vi "Initialise Listbox.vi"(8 "error in (no error)":errorcluster, 11 "MulticolumnListbox in":refnum<vi>) -> (0 "error out":errorcluster)   [LabVIEW 2016, in "Assert API Components.lvlib" / "Assert Display.lvlib" / "Main Display.lvlib" / "Main Display.lvclass"]
uses:
  Main Display.lvclass
  <vilib>/Utility/miscctls.llb/LVRowAndColumnTypeDef.ctl
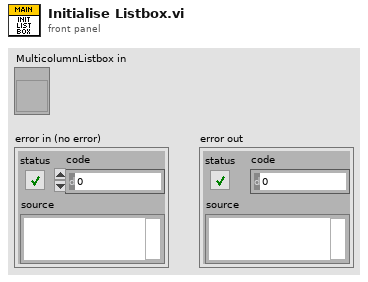
[diagram p1: front panel]
types:
  T1 = typedef "LVRowAndColumnTypeDef.ctl" = cluster{"Row":i32, "Column":i32}
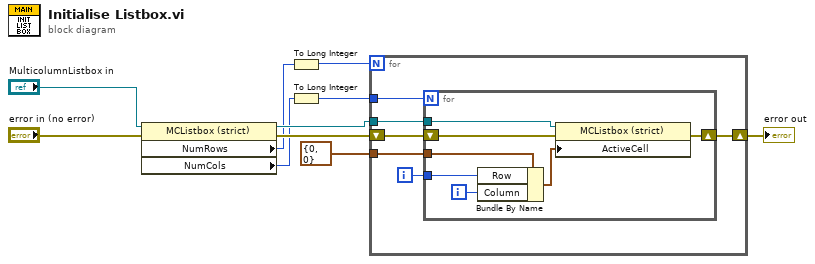
[diagram p0: block diagram]
diagram:
  n1 = property class="MCListbox (strict)"(reference="MulticolumnListbox in", error in="error in (no error)") -> (reference out=w6:refnum<vi>, error out=w9:errorcluster, "NumRows"=w4:u32, "NumCols"=w3:u32)
  n2 = To Long Integer(number=w4) -> (32bit integer=w2:i32)
  n3 = To Long Integer(number=w3) -> (32bit integer=w1:i32)
  n4 = for {
    N: w2 -> [_]
    tunnel: w6 -> [w14]
    shift-right: [w15] -> w7
    shift-left: w9 -> [w16]
    tunnel: T1 {"Row"=0, "Column"=0} ("Active Cell:Active Cell") -> [w13]
    tunnel: w1 -> [w12]
    i -> [w11]
    n5 = for {
      N: w12 -> [_]
      tunnel: w14 -> [w21]
      shift-right: [w22] -> w15
      shift-left: w16 -> [w23]
      tunnel: w13 -> [w20]
      tunnel: w11 -> [w17]
      i -> [w18]
      n6 = Bundle By Name(cluster=w20, "Row"=w17, "Column"=w18) -> (w19:T1)
      n7 = property class="MCListbox (strict)"(reference=w21, error in=w23, "ActiveCell"=w19) -> (error out=w22:errorcluster)  [unwired: 1 out]
    }
  }
  "error out" <- w7
